vi "XIPIN_Divider_Generator_5_1.vi"   [LabVIEW 2017]
doc: "This core provides division using one of three algorithms. The LUT-Mult algorithm is suitable for very small operands. The Radix-2 algorithm provides a solution suitable for small to medium operand division, and High Radix algorithm provides a solution based upon XtremeDSP slices and so is well suited to larger operands (that is, above about 16 bits wide).\n------------------------------------\n<b>Need License</b> : No\n<b>Interface</b> : AXI4-Stream"
uses:
  <vilib>/rvi/XilinxIP/XIPIN_XNode/niFpgaXIPIN.xnode
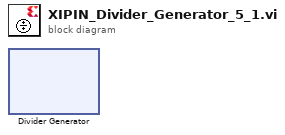
[diagram p0: block diagram]
diagram:
  n1 = xnode ("Divider Generator")() -> ()
